vi "TestStand - Insert element  into  1D Array.vi"(0 "Sequence Context":refnum<k7>, 2 "Lookup String":string="Locals.NumericArray", 5 "Data In":dbl, 11 "Error In":errorcluster) -> (15 "Error Out":errorcluster)   [LabVIEW 2013]
doc: "This VI inserts 1D array into TestStand 1D Array"
uses:
  <vilib>/addons/TestStand/_TSUtility.llb/TestStand - Get Property Value (Numeric Array).vi
  <vilib>/addons/TestStand/_TSUtility.llb/TestStand - Set Property Value (Numeric Array).vi
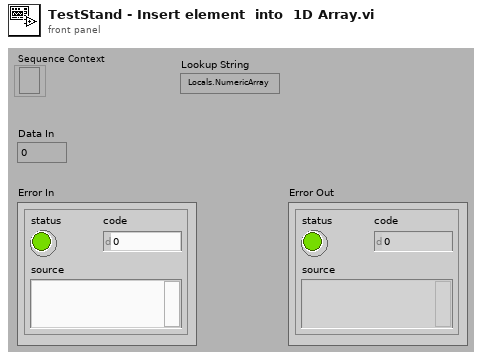
[diagram p1: front panel]
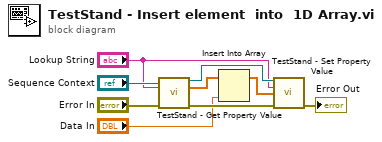
[diagram p0: block diagram]
diagram:
  n1 = call-poly <vilib>:"TestStand - Get Property Value.vi"("Sequence Context In"="Sequence Context", "Lookup String"="Lookup String", "error in (no error)"="Error In") -> ("Sequence Context Out"=w7:refnum<k7>, "Value"=w5:dbl[], "error out"=w8:errorcluster)  [unwired: 10 out]
  n2 = Insert Into Array(array=w5, new element="Data In") -> (w4:dbl[])  [unwired: 1 in]
  n3 = call-poly <vilib>:"TestStand - Set Property Value.vi"("Sequence Context In"=w7, "Lookup String"="Lookup String", "New Value"=w4, "error in (no error)"=w8) -> ("error out"=→"Error Out":errorcluster)  [unwired: 1 in, 10 out]
